vi "Experiment_description.vi"() -> (0 "Canceled":bool, 3 "Process conditions":T1)   [LabVIEW 2012]
uses:
  Controls/process condition.ctl
panel:
  in  "Save":bool
  in  "Cancel options":bool
  in  "Operator":string caption="Оператор"
  in  "Electrolyte composition":string[][](table)=[["KOH", "2"], ["Жидкое стекло", "9"]] caption="Состав электролита"
  in  "Purpose":string caption="Цель исследования"
  in  "Alloy":string caption="Сплав"
  in  "Clear":bool
  in  "MDO_mode":string(combo)="ПОЭП" caption="Режим работы"
  in  "Bath volume":string(combo)="30 л" caption="Ванна"
  in  "MDO duration":i32 caption="Длительность"
  # "Описание эксперимента"
  # "мин"
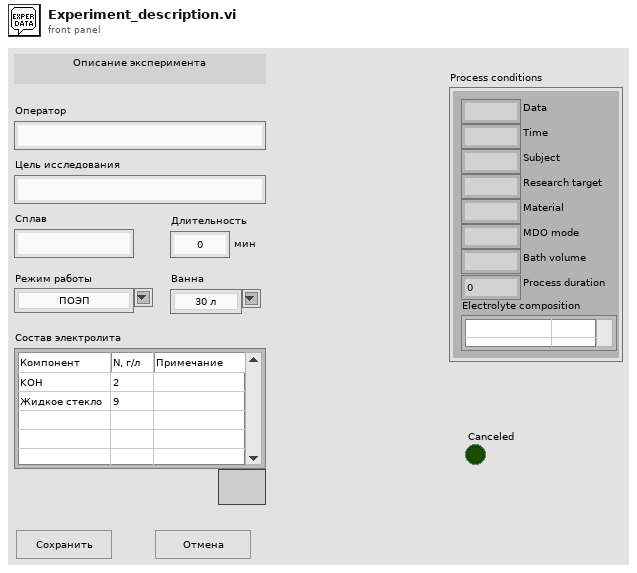
[diagram p1: front panel]
types:
  T1 = typedef "process condition.ctl" = cluster{"Data":string, "Time":string, "Subject":string, "Research target":string, "Material":string, "Electrolyte composition":string[][], "MDO mode":string, "Bath volume":string, "Process duration":i32}
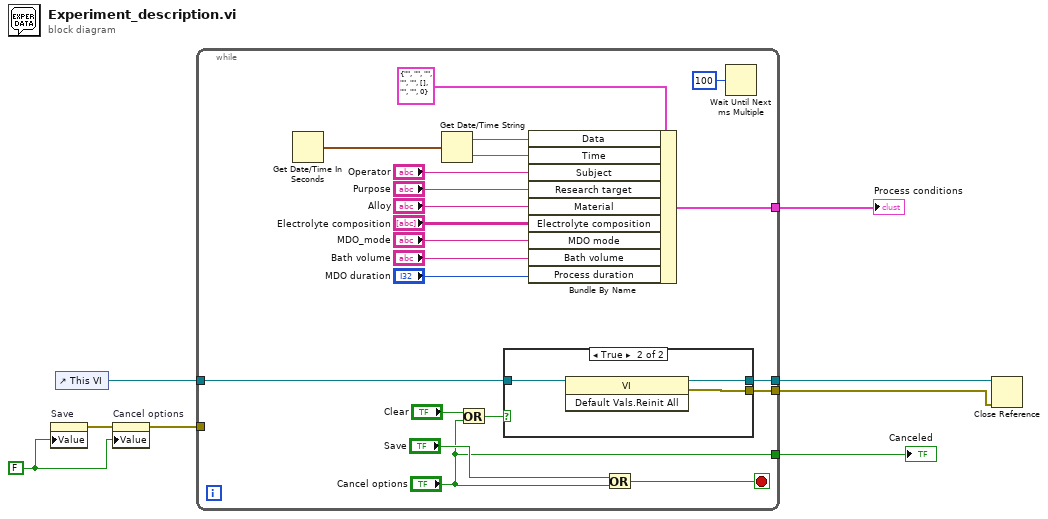
[diagram p0: block diagram]
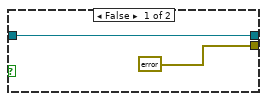
[diagram p2: hidden frame]
diagram:
  w4 = FALSE ("Save")
  n1 = property on="Save" class="Bool (strict)"("Value"=w4) -> (error out=w6:errorcluster)  [unwired: 2 in, 1 out]
  n2 = control-ref of="This VI"() -> (w8:refnum<vi>)
  n3 = property on="Cancel options" class="Bool (strict)"(error in=w6, "Value"=w4) -> (error out=w5:errorcluster)  [unwired: 1 in, 1 out]
  n4 = while {
    tunnel: w8 -> [w28]
    tunnel: [w27] -> w2
    tunnel: [w26] -> w1
    tunnel: [w20] -> w7
    tunnel: w5 -> [_]
    tunnel: ["Cancel options"] -> w3
    stop <- w24 stop-if-true
    n5 = Get Date/Time In Seconds() -> (seconds since 1Jan1904=w10:timestamp)
    n6 = Get Date/Time String(seconds (now)=w10) -> (date string=w12:string, time string=w11:string)  [unwired: 2 in]
    n7 = Or(x="Clear", y="Cancel options") -> (x .or. y?=w22:bool)
    n8 = case shown="True" w22 {
      tunnel: w28 -> [w31 w34]
      tunnel: [w31 w33] -> w27
      tunnel: [errorcluster {"status"=FALSE, "code"=0, "source"=""} ("error out") w32] -> w26
      frame False {
      }
      frame True {
        n9 = invoke class="VI" method="Default Vals.Reinit All"(reference=w34) -> (reference out=w33:refnum<vi>, error out=w32:errorcluster)  [unwired: 2 in, 1 out]
      }
    }
    n10 = Bundle By Name(cluster=T1 {"Data"="", "Time"="", "Subject"="", "Research target"="", "Material"="", "Electrolyte composition"=[], "MDO mode"="", "Bath volume"="", "Process duration"=0} ("Process conditions"), "Data"=w12, "Time"=w11, "Subject"="Operator", "Research target"="Purpose", "Material"="Alloy", "Electrolyte composition"="Electrolyte composition", "MDO mode"="MDO_mode", "Bath volume"="Bath volume", "Process duration"="MDO duration") -> (w20:T1)
    n11 = Or(x="Save", y="Cancel options") -> (x .or. y?=w24:bool)
    n12 = Wait Until Next ms Multiple(millisecond multiple=u32 100) -> ()  [unwired: 1 out]
  }
  "Canceled" <- w3
  "Process conditions" <- w7
  n13 = Close Reference(reference=w2, error in (no error)=w1) -> ()  [unwired: 1 out]
